vi "getContext.vi"(0 "instruction target in":refnum<class "niInstr Instruction Target v1 Host.lvclass">, 5 "instance":u8, 11 "error in":errorcluster) -> (4 "Interface":T1, 15 "error out":errorcluster)   [LabVIEW 2017, in "ThreePhasePLLInterface.lvlib"]
uses:
  ThreePhasePLLInterface.lvlib
  <instrlib>/_niInstr/Instruction Framework/v1/Host/Instruction Target/niInstr Instruction Target v1 Host.lvclass
  InterfaceRef.ctl
  <instrlib>/_niInstr/Instruction Framework/v1/Host/Instruction Framework Context/niInstr Instruction Framework Context v1 Host.lvclass
  <vilib>/NI/PowerElectronicsControl/ActiveFrontEnd/AFE_Interface/InterfaceRef.ctl
  <instrlib>/_niInstr/Instruction Framework/v1/Host/Subsystem Map/Private/Lookup Single Context.vi
  <instrlib>/_niInstr/Instruction Framework/v1/Host/Subsystem Map/niInstr Subsystem Map v1 Host.lvclass
  <vilib>/NI/PowerElectronicsControl/ActiveFrontEnd/AFE_Interface/AFE_interface.lvlib
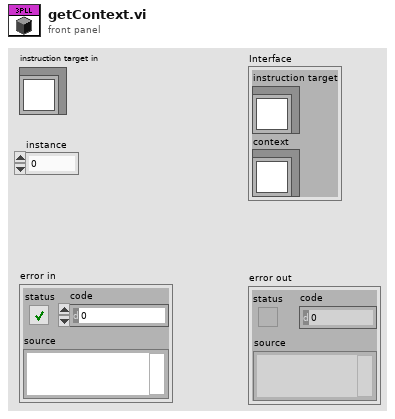
[diagram p1: front panel]
types:
  T1 = typedef "ThreePhasePLLInterface.lvlib/InterfaceRef.ctl" = cluster{"instruction target":refnum<class "niInstr Instruction Target v1 Host.lvclass">, "context":refnum<class "niInstr Instruction Framework Context v1 Host.lvclass">}
  T2 = typedef "AFE_interface.lvlib/InterfaceRef.ctl" = cluster{"instruction target":refnum<class "niInstr Instruction Target v1 Host.lvclass">, "context":refnum<class "niInstr Instruction Framework Context v1 Host.lvclass">}
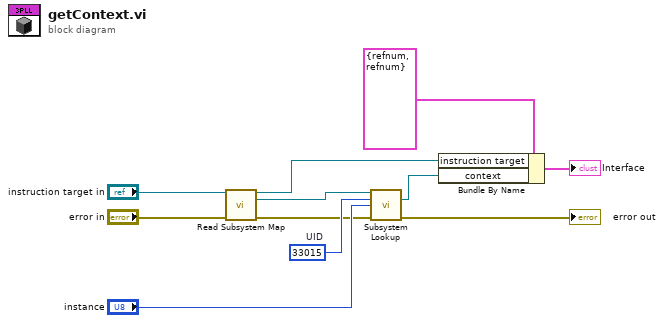
[diagram p0: block diagram]
diagram:
  w11 = u16 33015  # UID
  n1 = call <instrlib>:"Read Subsystem Map.vi"("instruction target in"="instruction target in", "error in"="error in") -> ("instruction target out"=w2:refnum<class "niInstr Instruction Target v1 Host.lvclass">, "subsystem map"=w8:refnum<class "niInstr Subsystem Map v1 Host.lvclass">, "error out"=w9:errorcluster)  [unwired: 11 in]
  n2 = call-poly <instrlib>:"Subsystem Lookup.vi"("subsystem map in"=w8, "UID"=w11, "instance"="instance", "error in"=w9) -> ("context"=w3:refnum<class "niInstr Instruction Framework Context v1 Host.lvclass">, "error out"=→"error out":errorcluster)  [unwired: 8 in, 2 out]
  n3 = Bundle By Name(cluster=T2 {"instruction target"=refnum, "context"=refnum} ("Interface"), "instruction target"=w2, "context"=w3) -> (→"Interface":T2)
